vi "Frame Loop if Necessary.vi"(8 "error in (no error)":errorcluster, 11 "Video File in":refnum<class "Video File.lvclass">) -> (0 "error out":errorcluster, 1 "Looped?":bool, 2 "Finished?":bool, 3 "Video File out":refnum<class "Video File.lvclass">)   [LabVIEW 2018, in "Video File.lvclass"]
uses:
  Video File.lvclass
  Video File.lvclass/Video File.ctl
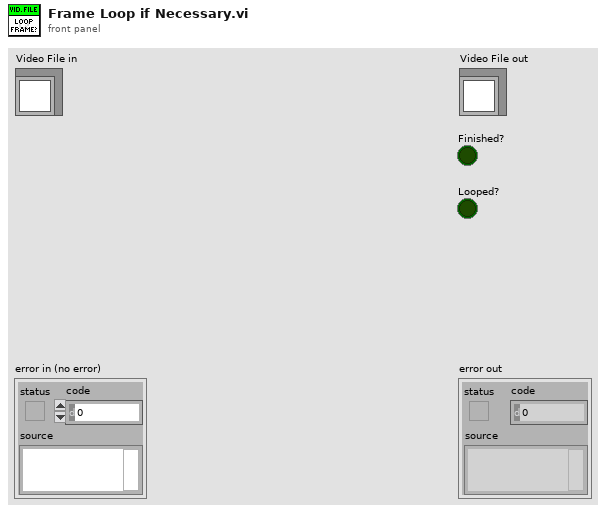
[diagram p1: front panel]
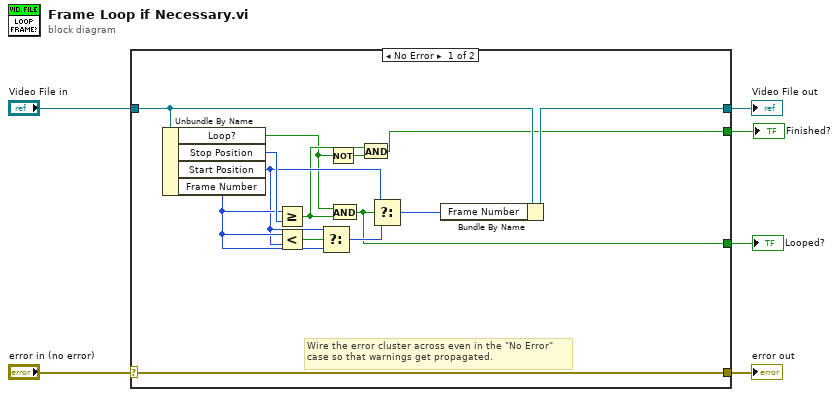
[diagram p0: block diagram]
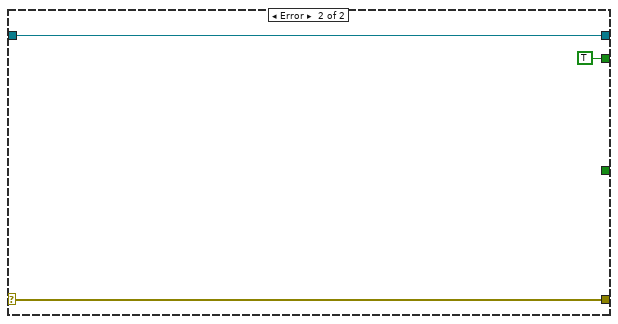
[diagram p2: hidden frame]
diagram:
  n1 = case shown="No Error" "error in (no error)" {
    selector: "error in (no error)" -> [w20 w23]
    tunnel: [w20 w23] -> w5
    tunnel: [w18 w22] -> w3
    tunnel: "Video File in" -> [w19 w22]
    tunnel: [w7 TRUE] -> w2
    tunnel: [w8 _] -> w1
    frame No Error {
      # "Wire the error cluster across even in the \"No Error\"\ncase so that warnings get propagated."
      n2 = Unbundle By Name(w19) -> ("Loop?"=w10:bool, "Stop Position"=w17:u32, "Start Position"=w14:u32, "Frame Number"=w15:u32)
      n3 = Greater Or Equal?(x=w15, y=w17) -> (x >= y?=w11:bool)
      n4 = Less?(x=w15, y=w14) -> (x < y?=w16:bool)
      n5 = Select(t=w14, s=w16, f=w15) -> (s? t:f=w13:u32)
      n6 = Not(x=w10) -> (.not. x?=w9:bool)
      n7 = And(x=w10, y=w11) -> (x .and. y?=w8:bool)
      n8 = And(x=w11, y=w9) -> (x .and. y?=w7:bool)
      n9 = Select(t=w14, s=w8, f=w13) -> (s? t:f=w12:u32)
      n10 = Bundle By Name(cluster=w19, "Frame Number"=w12) -> (w18:refnum<class "Video File.lvclass">)
    }
    frame Error {
    }
  }
  "error out" <- w5
  "Video File out" <- w3
  "Finished?" <- w2
  "Looped?" <- w1
